vi "String NotEQ.vi"(11 "Data In":string) -> (3 "Data Out":string)   [LabVIEW 2016]
uses:
  Core/Assert API Components/Failure Actions.ctl
  Core/Assert API Components/Assert API Components.lvlib
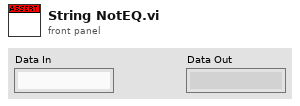
[diagram p1: front panel]
types:
  T1 = typedef "Assert API Components.lvlib/Failure Actions.ctl" = enum16{"None", "Log To File", "Pause Execution", "Abort Execution"}
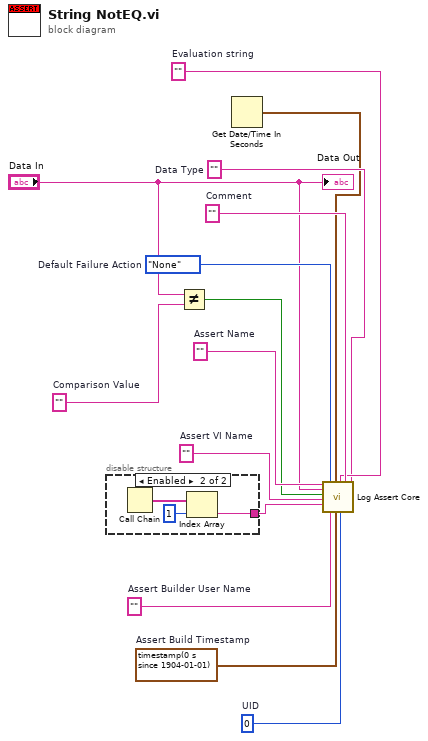
[diagram p0: block diagram]
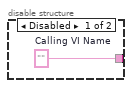
[diagram p2: hidden frame]
diagram:
  w2 = 0  # UID
  w4 = ""  # Assert VI Name
  w5 = ""  # Assert Builder User Name
  w6 = timestamp(0 s since 1904-01-01)  # Assert Build Timestamp
  w7 = ""  # Data Type
  w11 = ""  # Comment
  w8 = ""  # Evaluation string
  w13 = Failure_Actions."None"  # Default Failure Action
  w14 = ""  # Assert Name
  w12 = ""  # Comparison Value
  n1 = disable-structure shown="Enabled" {
    disable-tunnel: [w15 w16] -> w1
    frame Disabled {
      w15 = ""  # Calling VI Name
    }
    frame Enabled {
      n2 = Call Chain() -> (call chain=w17:string[])
      n3 = Index Array(array=w17, index=1) -> (element=w16:string)
    }
  }
  n4 = Not Equal?(x="Data In", y=w12) -> (x != y?=w9:bool)
  n5 = Get Date/Time In Seconds() -> (seconds since 1Jan1904=w3:timestamp)
  n6 = call "Log Assert Core.vi"("Assert Name"=w14, "Data Value"="Data In", "Status"=w9, "Assert VI Name"=w4, "Calling VI Name"=w1, "Failure Action"=w13, "Assert Builder User Name"=w5, "Last Update"=w3, "Assert Build Timestamp"=w6, "Evaluation String"=w8, "Assert VI UID"=w2, "Comment"=w11, "Data Type"=w7) -> ()  [unwired: 7 in]
  "Data Out" <- "Data In"
